vi "Read Time.vi"(8 "error in (no error)":errorcluster, 11 "ExtFlatShutt in":refnum<class "ExtFlatShutt.lvclass">) -> (0 "error out":errorcluster, 2 "Time Stamp":timestamp, 3 "ExtFlatShutt out":refnum<class "ExtFlatShutt.lvclass">)   [LabVIEW 2016, in "ExtFlatShutt.lvclass"]
uses:
  ExtFlatShutt.lvclass
  Shutter.lvclass
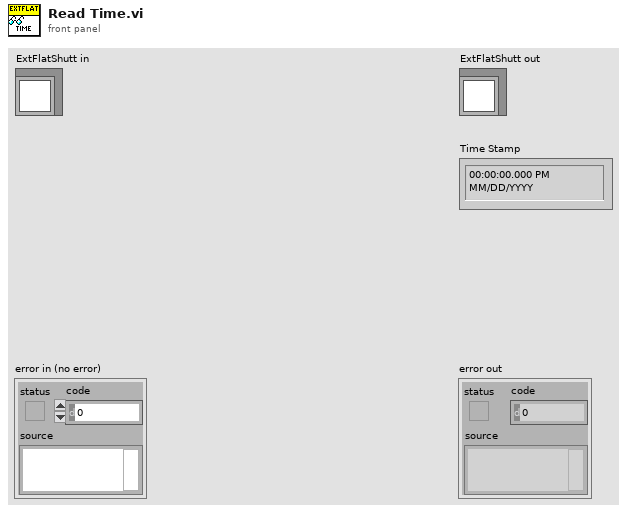
[diagram p1: front panel]
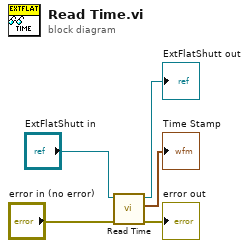
[diagram p0: block diagram]
diagram:
  n1 = call-parent "Read Time.vi"("error in (no error)"="error in (no error)", "Shutter in"="ExtFlatShutt in") -> ("error out"=→"error out":errorcluster, "Time Stamp"=→"Time Stamp":timestamp, "Shutter out"=→"ExtFlatShutt out":refnum<class "ExtFlatShutt.lvclass">)  [unwired: 7 in]
